vi "MKS CTLR - Save Data.vi"(0 "Array":dbl[](array[numeric]), 1 "Save Data to File":bool, 2 "Ext time (sec)":dbl format="%#_10g") -> (3 "Current time (sec)":dbl format="%#_10g")   [LabVIEW 2013]
uses:
  <vilib>/Utility/file.llb/Write To Spreadsheet File (string).vi
  <vilib>/Utility/file.llb/Write To Spreadsheet File (DBL).vi
panel:
  out "Day":string
  out "Appended array":dbl[](array[numeric]) format="%#_10g"
  out "File name":string
  # "Saves data to spreadsheet file"
  # "Creates file with name including current time\nand header plus data"
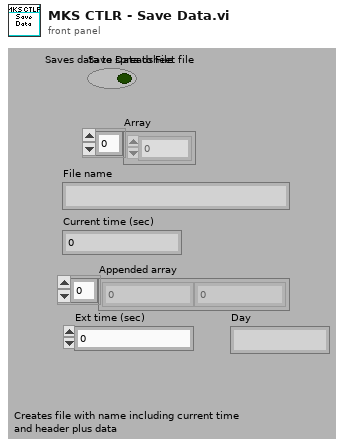
[diagram p1: front panel]
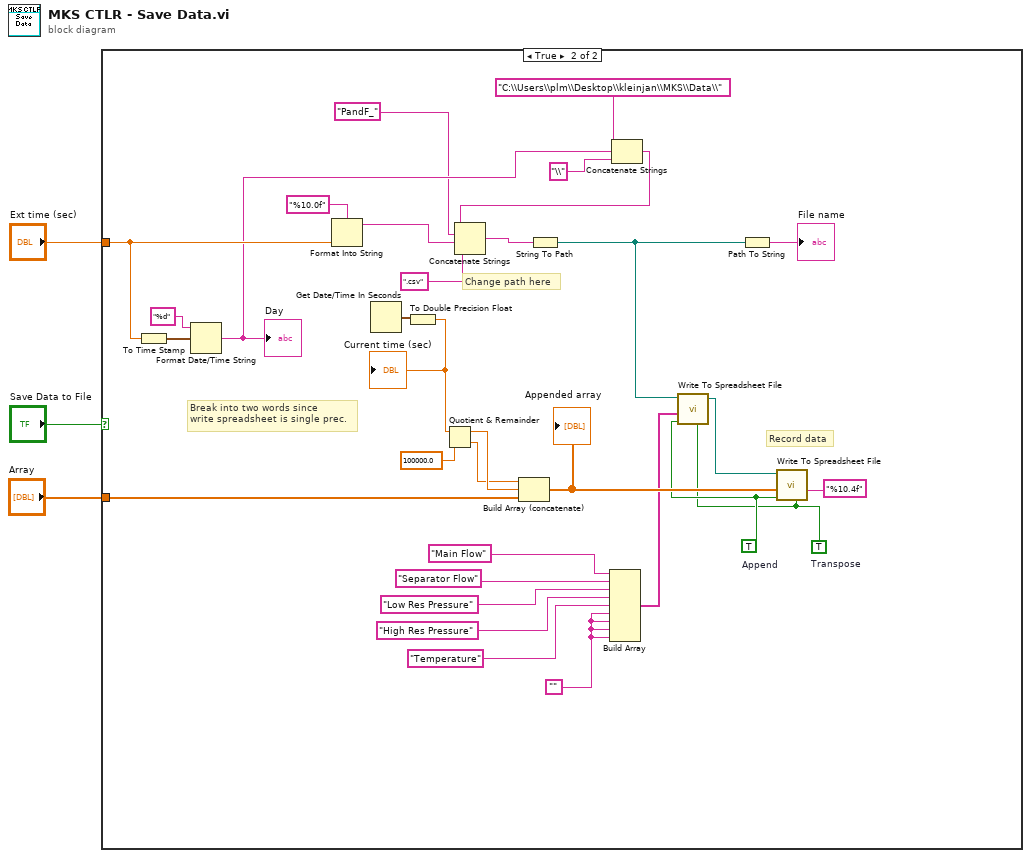
[diagram p0: block diagram]
diagram:
  n1 = case shown="True" "Save Data to File" {
    tunnel: "Array" -> [_ w4]
    tunnel: "Ext time (sec)" -> [_ w18]
    frame False {
      # "Not writing file"
    }
    frame True {
      w5 = ""
      w20 = TRUE  # Append
      w19 = TRUE  # Transpose
      # "Change path here"
      # "Record data"
      # "Break into two words since\nwrite spreadsheet is single prec."
      n2 = To Time Stamp(1:w18) -> (0:w17:timestamp)
      n3 = Format Date/Time String(time format string (%c)="%d", seconds (now)=w17) -> (date/time string=w14:string)  [unwired: 1 in]
      "Day" <- w14
      n4 = Format Into String "Format Into String"(format string="%10.0f", w18) -> (resulting string=w34:string)  [unwired: 2 in, 1 out]
      n5 = Get Date/Time In Seconds() -> (seconds since 1Jan1904=w30:timestamp)
      n6 = To Double Precision Float(number=w30) -> (double precision float=w28:dbl)
      "Current time (sec)" <- w28
      n7 = Quotient & Remainder(x=w28, y=100000.0) -> (x-y*floor(x/y)=w27:dbl, floor(x/y)=w25:dbl)
      n8 = Build Array (concatenate) "Build Array"(w25, w27, w4) -> (w29:dbl[])
      "Appended array" <- w29
      n9 = Build Array("Main Flow" ("element"), "Separator Flow" ("element"), "Low Res Pressure" ("element"), "High Res Pressure" ("element"), "Temperature" ("element"), w5, w5, w5, w5) -> (w21:string[])
      n10 = Concatenate Strings("C:\\Users\\plm\\Desktop\\kleinjan\\MKS\\Data\\", w14, "\\") -> (w12:string)
      n11 = Concatenate Strings(w12, "PandF_" ("string"), w34, ".csv") -> (w32:string)
      n12 = String To Path(string=w32) -> (path=w23:path)
      n13 = call-poly <vilib>:"Write To Spreadsheet File.vi"("transpose? (no:F)"=w19, "append to file? (new file:F)"=w20, "1D data"=w21, "file path (dialog if empty)"=w23) -> ("new file path (Not A Path if cancelled)"=w22:path)  [unwired: 4 in]
      n14 = Path To String(path=w23) -> (string=→"File name":string)
      n15 = call-poly <vilib>:"Write To Spreadsheet File.vi"("transpose? (no:F)"=w19, "format (%.3f)"="%10.4f", "append to file? (new file:F)"=w20, "1D data"=w29, "file path (dialog if empty)"=w22) -> ()  [unwired: 3 in, 1 out]
    }
  }
